vi "FTW-ERR-ThrowConditionalWarning.vi"(7 "Warning Message":string, 9 "Error Code":i32, 11 "error in":errorcluster, 12 "Throw?":bool, 13 "Source Level":i32 caption="Source Level (0 = This VI's caller)") -> (15 "error out":errorcluster)   [LabVIEW 2018]
doc: "Throws an error if the \"Error Code\" input is non-zero."
panel:
  # "Inputs"
  # "Outputs"
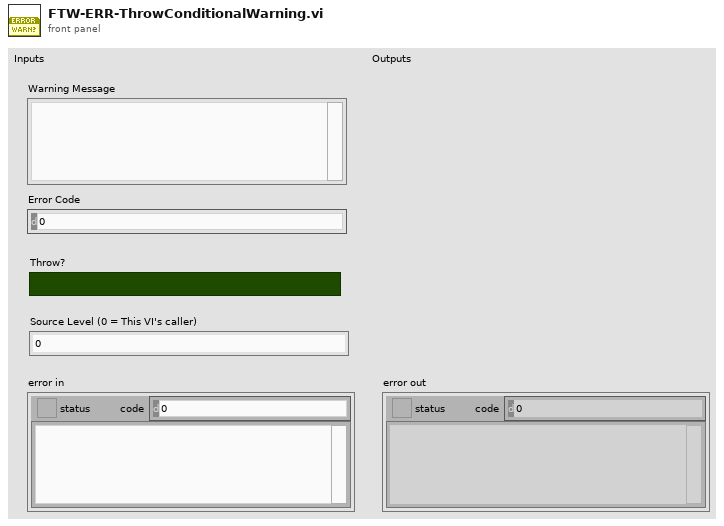
[diagram p1: front panel]
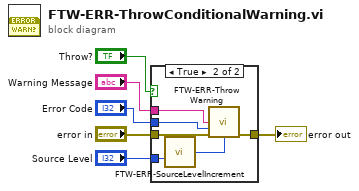
[diagram p0: block diagram]
diagram:
  n1 = case shown="True" "Throw?" {
    tunnel: "error in" -> [w7 w9]
    tunnel: "Warning Message" -> [_ w11]
    tunnel: "Error Code" -> [_ w12]
    tunnel: [w7 w10] -> w3
    tunnel: "Source Level" -> [_ w13]
    frame False {
    }
    frame True {
      n2 = call "FTW-ERR-SourceLevelIncrement.vi"("SourceLevelIn"=w13) -> ("SourceLevelOut"=w8:i32)
      n3 = call "FTW-ERR-ThrowWarning.vi"("Warning Message"=w11, "Error Code"=w12, "error in"=w9, "Source Level"=w8) -> ("error out"=w10:errorcluster)  [unwired: 11 in]
    }
  }
  "error out" <- w3
